vi "HEWH Read All MW100 Inputs.vi"(0 "MW100":refnum<visa-resource-name>="MW100", 1 "LV Program":T1, 11 "Error In":errorcluster) -> (4 "MW100 Output":refnum<visa-resource-name>, 6 "MW100 Data Cluster Output":T4, 10 "PowerData":T3, 14 "Tank Display":dbl[](array[numeric]), 15 "Error Out":errorcluster)   [LabVIEW 2016]
uses:
  Type Definitions/HEWH MW100 Data Cluster.ctl
  Type Definitions/HEWH Power Data.ctl
  MW100/Type Definitions/HEWH MW100 Channel Numbers.ctl
  Utility/Save File/File Setup (Public)/Type Definition/Save File DOE LabView Program.ctl
  Utility/Save File/File Setup.lvlib
panel:
  in  "HEWH MW100 Channel Numbers 2":T2="A010"
  in  "HEWH MW100 Channel Numbers":T2="011"
  in  "MW100 Data Cluster":T4
  out "Data (Label, Channel, Data)":string[][](array[string])
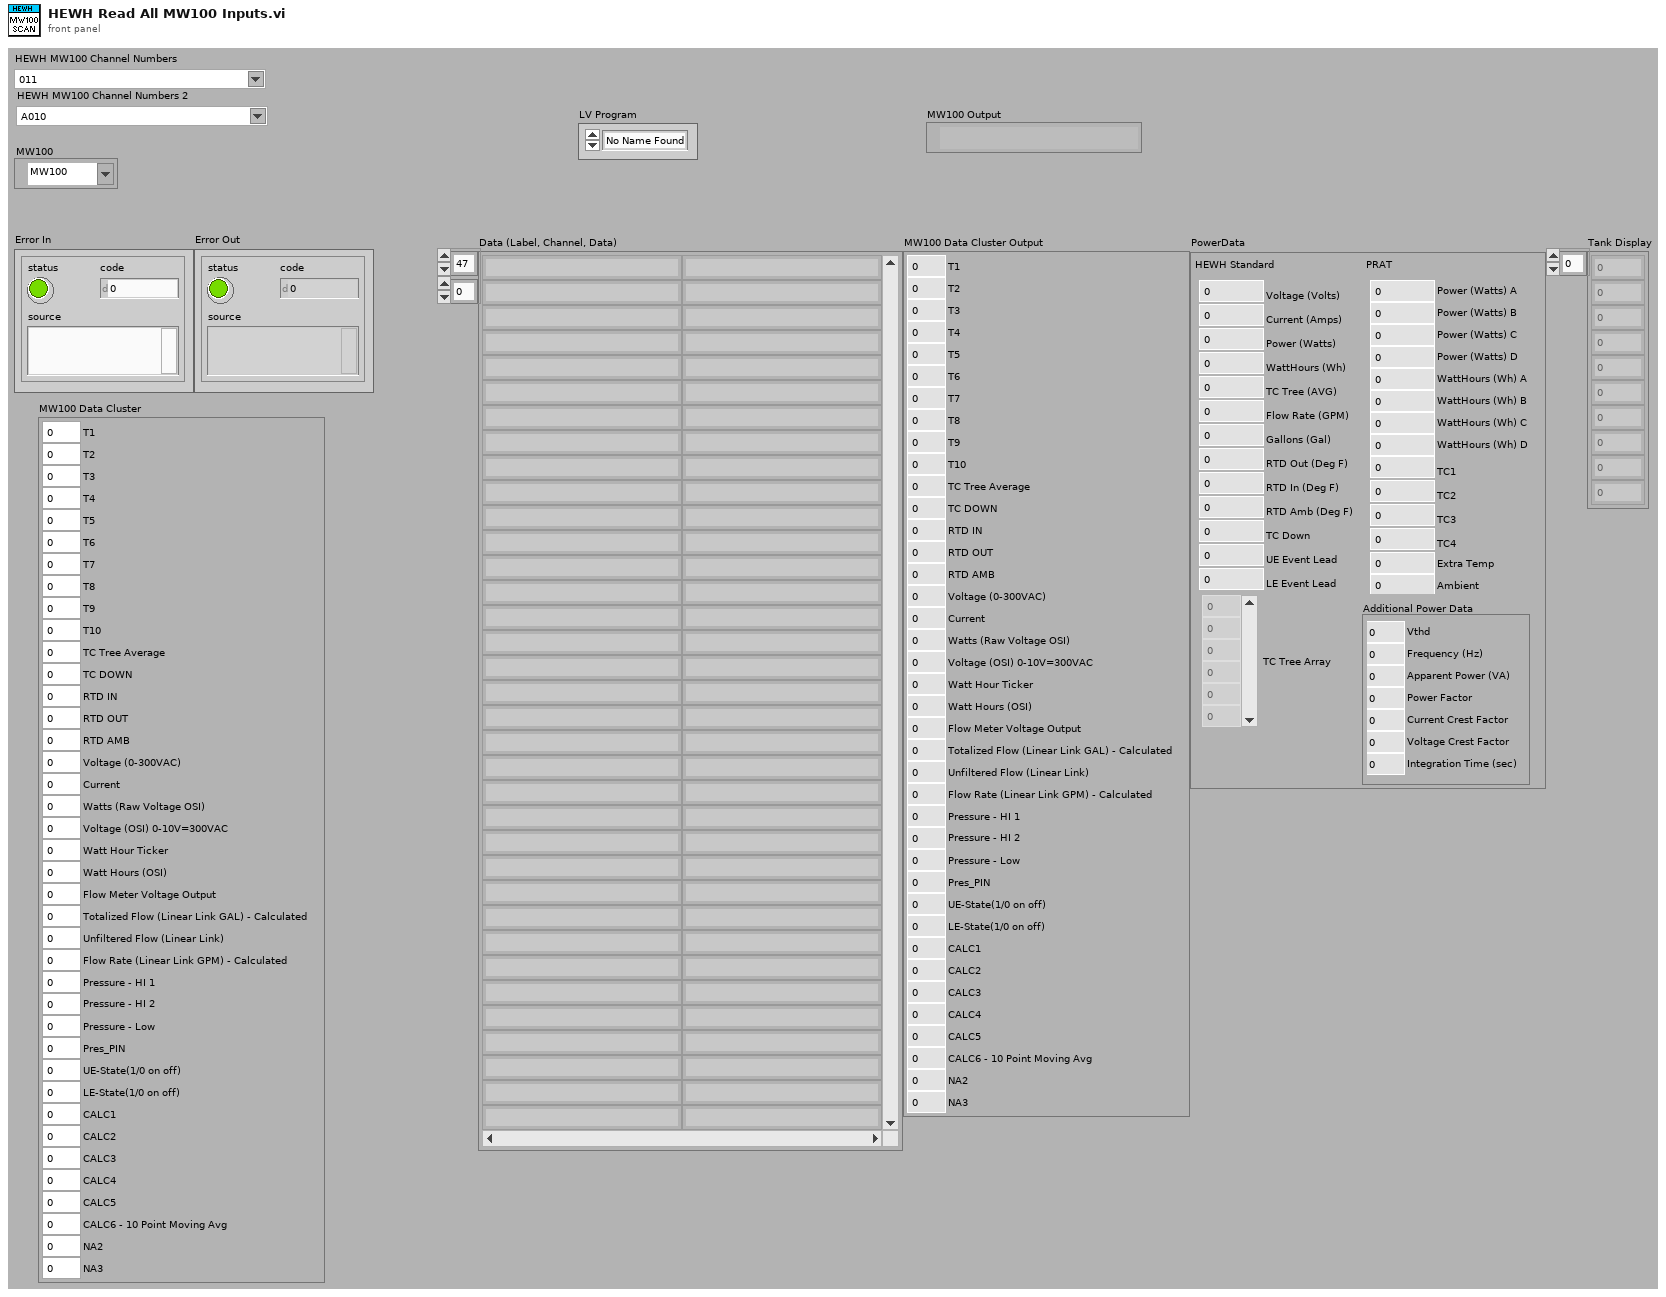
[diagram p1: front panel]
types:
  T1 = typedef "File Setup.lvlib/Save File DOE LabView Program.ctl" = enum16{"No Name Found", "DOE Stand", "Dishwasher Kitchen", "Portable Stand", "HEWH", "Dryer", "Dryer WILT", "HCC", "PRAT", "HEWH RLT", "Refrigeration"}
  T2 = typedef "HEWH MW100 Channel Numbers.ctl" = string
  T3 = typedef "HEWH Power Data.ctl" = cluster{"HEWH Standard":cluster{"Voltage (Volts)":dbl, "Current (Amps)":dbl, "Power (Watts)":dbl, "WattHours (Wh)":dbl, "TC Tree (AVG)":dbl, "Flow Rate (GPM)":dbl, "Gallons (Gal)":dbl, "RTD Out (Deg F)":dbl, "RTD In (Deg F)":dbl, "RTD Amb (Deg F)":dbl, "TC Down":dbl, "UE Event Lead":i32, "LE Event Lead":i32, "TC Tree Array":dbl[]}, "PRAT":cluster{"Power (Watts) A":dbl, "Power (Watts) B":dbl, "Power (Watts) C":dbl, "Power (Watts) D":dbl, "TC1":dbl, "TC2":dbl, "TC3":dbl, "TC4":dbl, "WattHours (Wh) A":dbl, "WattHours (Wh) B":dbl, "WattHours (Wh) C":dbl, "WattHours (Wh) D":dbl, "Ambient":dbl, "Extra Temp":dbl}, "Additional Power Data":cluster{"Vthd":dbl, "Frequency (Hz)":dbl, "Apparent Power (VA)":dbl, "Power Factor":dbl, "Current Crest Factor":dbl, "Voltage Crest Factor":dbl, "Integration Time (sec)":dbl}}
  T4 = typedef "HEWH MW100 Data Cluster.ctl" = cluster{"T1":dbl, "T2":dbl, "T3":dbl, "T4":dbl, "T5":dbl, "T6":dbl, "T7":dbl, "T8":dbl, "T9":dbl, "T10":dbl, "TC Tree Average":dbl, "TC DOWN":dbl, "RTD IN":dbl, "RTD OUT":dbl, "RTD AMB":dbl, "Voltage (0-300VAC)":dbl, "Current":dbl, "Watts (Raw Voltage OSI)":dbl, "Voltage (OSI) 0-10V=300VAC":dbl, "Watt Hour Ticker":dbl, "Watt Hours (OSI)":dbl, "Flow Meter Voltage Output":dbl, "Totalized Flow (Linear Link GAL) - Calculated":dbl, "Unfiltered Flow (Linear Link)":dbl, "Flow Rate (Linear Link GPM) - Calculated":dbl, "Pressure - HI 1":dbl, "Pressure - HI 2":dbl, "Pressure - Low":dbl, "Pres_PIN":dbl, "UE-State(1/0 on off)":dbl, "LE-State(1/0 on off)":dbl, "CALC1":dbl, "CALC2":dbl, "CALC3":dbl, "CALC4":dbl, "CALC5":dbl, "CALC6 - 10 Point Moving Avg":dbl, "NA2":dbl, "NA3":dbl}
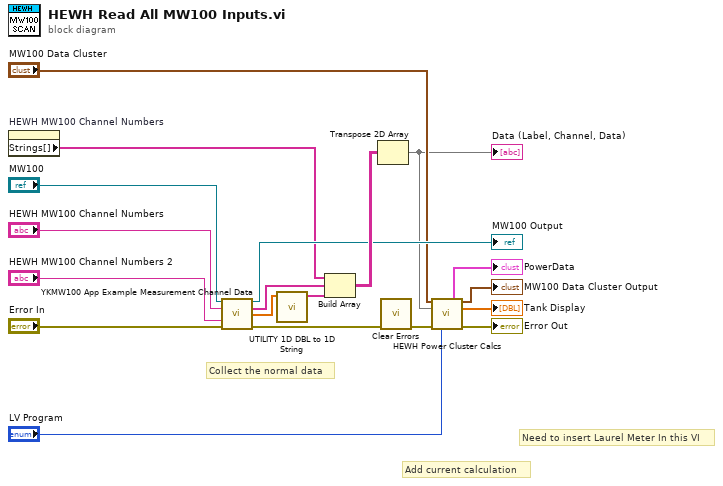
[diagram p0: block diagram]
diagram:
  # "Need to insert Laurel Meter In this VI"
  # "Add current calculation"
  # "Collect the normal data"
  n1 = property on="HEWH MW100 Channel Numbers" class="CmbBox (strict)"() -> ("Strings[]"=w11:string[])  [unwired: 2 in, 2 out]
  n2 = call "YKMW100 App Example Measurement Channel Data.vi"("VISA session"="MW100", "Start Channel (001)"="HEWH MW100 Channel Numbers", "End Channel (001)"="HEWH MW100 Channel Numbers 2", "error in (no error)"="Error In") -> ("dup VISA session"=→"MW100 Output":refnum<visa-resource-name>, "Channel List"=w18:string[], "Data List"=w6:dbl[], "error out"=w4:errorcluster)  [unwired: 4 in, 4 out]
  n3 = call "UTILITY 1D DBL to 1D String.vi"("1D DBL"=w6) -> ("1D String"=w5:string[])  [unwired: 10 in]
  n4 = Build Array(w11, w18, w5) -> (w17:string[][])
  n5 = Transpose 2D Array(2D array=w17) -> (transposed array=w9:string[][])
  "Data (Label, Channel, Data)" <- w9
  n6 = call <vilib>:"Clear Errors.vi"("error in (no error)"=w4) -> ("error out"=w2:errorcluster)  [unwired: 5 in, 1 out]
  n7 = call "HEWH Power Cluster Calcs.vi"("MW100 Data Cluster"="MW100 Data Cluster", "Data (Label, Channel, Data)"=w9, "Error In"=w2, "LV Program"="LV Program") -> ("PowerData"=→"PowerData":T3, "MW100 Data Cluster Output"=→"MW100 Data Cluster Output":T4, "Tank Display"=→"Tank Display":dbl[], "Error Out"=→"Error Out":errorcluster)  [unwired: 8 in]
